vi "Reset ILC.vi"(0 "Model in":refnum<class "Model.lvclass">, 11 "error in (no error)":errorcluster) -> (4 "Model out":refnum<class "Model.lvclass">, 15 "error out":errorcluster)   [LabVIEW 2016, in "Model.lvclass"]
uses:
  Model.lvclass
  Modbus/DesktopModbus/DesktopModbus.lvclass
  common_rt_modbus/DynamicFrameParser/DynamicFrameParser.lvclass
  common_rt_ilc/ILC/ILC.lvclass
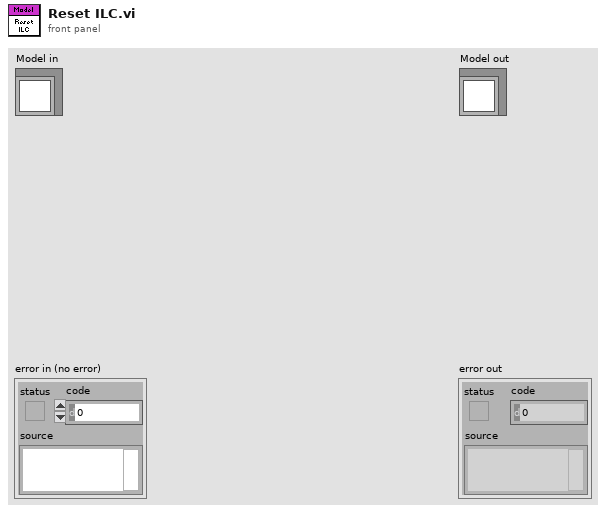
[diagram p1: front panel]
types:
  T1 = typedef "RTModbus.lvlib/TxFrame.ctl" = cluster{"Data":u8[], "WaitForTrigger":bool, "WaitForRx":u16, "TriggerIRQ":bool, "DelayMicroseconds":u16, "DelayMilliseconds":u16, "Timestamp":bool}
  T2 = typedef "RTModbus.lvlib/RxFrame.ctl" = cluster{"Data":u8[], "Timestamp":u64}
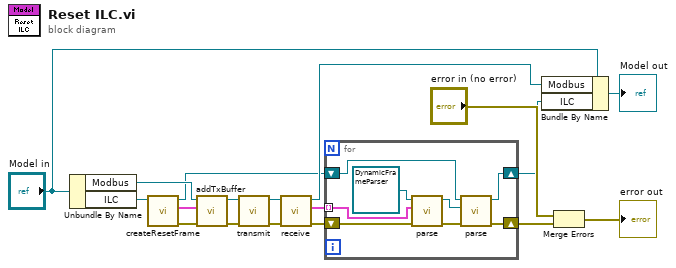
[diagram p0: block diagram]
diagram:
  n1 = Unbundle By Name("Model in") -> ("Modbus"=w17:refnum<class "DesktopModbus.lvclass">, "ILC"=w2:refnum<class "FAILC.lvclass">)
  n2 = call "createResetFrame.vi"("ILC in"=w2) -> ("error out"=w13:errorcluster, "TxFrame"=w16:T1, "ILC out"=w4:refnum<class "ILC.lvclass">)  [unwired: 8 in]
  n3 = call-dynamic "addTxBuffer.vi"("error in (no error)"=w13, "TxFrame"=w16, "DesktopModbus in"=w17) -> ("error out"=w12:errorcluster, "DesktopModbus out"=w15:refnum<class "DesktopModbus.lvclass">)  [unwired: 7 in]
  n4 = call-dynamic "transmit.vi"("error in (no error)"=w12, "DesktopModbus in"=w15) -> ("error out"=w11:errorcluster, "DesktopModbus out"=w14:refnum<class "DesktopModbus.lvclass">)  [unwired: 8 in]
  n5 = call-dynamic "receive.vi"("error in (no error)"=w11, "DesktopModbus in"=w14) -> ("error out"=w5:errorcluster, "Data"=w6:T2[], "DesktopModbus out"=w8:refnum<class "DesktopModbus.lvclass">)  [unwired: 7 in]
  n6 = for {
    tunnel: w6 -> [w24] mode=indexing
    shift-right: [w21] -> w3
    shift-left: w5 -> [w23]
    shift-right: [w19] -> w1
    shift-left: w4 -> [w20]
    n7 = call "parse.vi"("error in (no error)"=w23, "RxFrame"=w24, "FrameParser in"=refnum<class "DynamicFrameParser.lvclass"> refnum ("RTModbus.lvlib:DynamicFrameParser.lvclass")) -> ("error out"=w22:errorcluster, "FrameParser out"=w26:refnum<class "DynamicFrameParser.lvclass">)  [unwired: 7 in]
    n8 = call-dynamic "parse.vi"("error in (no error)"=w22, "DynamicFrameParser"=w26, "ILC in"=w20) -> ("error out"=w21:errorcluster, "ILC out"=w19:refnum<class "ILC.lvclass">)  [unwired: 6 in, 1 out]
  }
  n9 = Bundle By Name(cluster="Model in", "Modbus"=w8, "ILC"=w1) -> (→"Model out":refnum<class "Model.lvclass">)
  n10 = Merge Errors("error in (no error)", w3) -> (→"error out":errorcluster)
